vi "未命名 3 (子VI).vi"(10 "y输入":dbl, 11 "x":dbl) -> (3 "y输出":dbl)   [LabVIEW 2018]
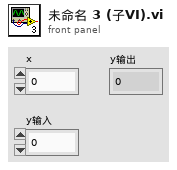
[diagram p1: front panel]
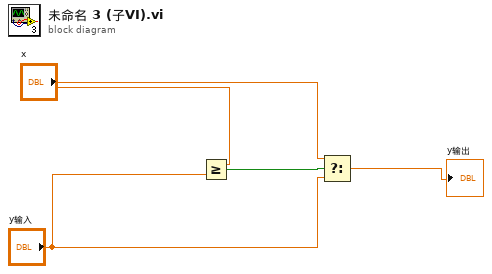
[diagram p0: block diagram]
diagram:
  n1 = Greater Or Equal?(x="x", y="y输入") -> (x >= y?=w1:bool)
  n2 = Select(t="x", s=w1, f="y输入") -> (s? t:f=→"y输出":dbl)
